vi "TestList.vi"() -> ()   [LabVIEW 2020]
uses:
  Redis_class/Redis.lvclass
panel:
  out "Connected?":bool
  out "Error Out":errorcluster
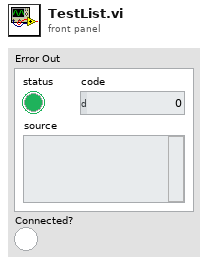
[diagram p1: front panel]
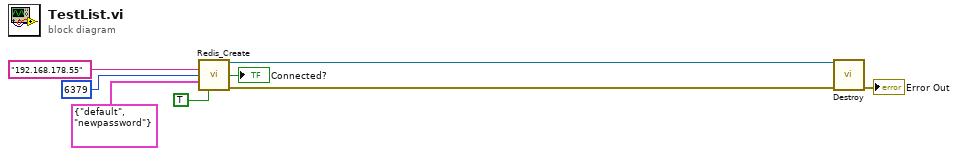
[diagram p0: block diagram]
diagram:
  n1 = call "Redis_Create.vi"("Host"="192.168.178.55", "Port"=u32 6379, "Authentication"=cluster{"Username":string, "Password":string} {"Username"="default", "Password"="newpassword"}, "UseAuthentication(F)"=TRUE) -> ("reference out"=w4:refnum<class "Redis.lvclass">, "Connected?"=→"Connected?":bool, "Error Out"=w5:errorcluster)  [unwired: 9 in]
  n2 = call-dynamic "Destroy.vi"("reference in"=w4, "Error In"=w5) -> ("Error Out"=→"Error Out":errorcluster)  [unwired: 12 in, 1 out]
